vi "SP Format Error Messages.vi"(8 "error in (no error)":errorcluster) -> (0 "error out":errorcluster)   [LabVIEW 2011]
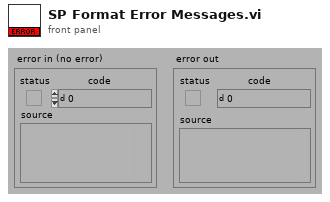
[diagram p1: front panel]
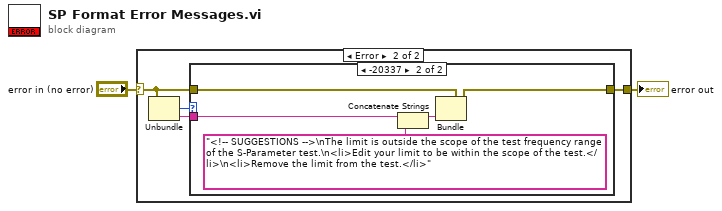
[diagram p0: block diagram]
diagram:
  n1 = case shown="Error" "error in (no error)" {
    selector: "error in (no error)" -> [w3 w5]
    tunnel: [w3 w4] -> w1
    frame No Error {
    }
    frame Error {
      n2 = Unbundle(w5) -> ("code"=w7:i32, "source"=w6:string)  [unwired: 1 out]
      n3 = case shown="-20337" w7 {
        tunnel: w6 -> [_ w13]
        tunnel: w5 -> [w8 w11]
        tunnel: [w8 w9] -> w4
        frame Default {
        }
        frame -20337 {
          n4 = Concatenate Strings(w13, "<!-- SUGGESTIONS -->\nThe limit is outside the scope of the test frequency range of the S-Parameter test.\n<li>Edit your limit to be within the scope of the test.</li>\n<li>Remove the limit from the test.</li>" ("string")) -> (w10:string)
          n5 = Bundle(cluster=w11, "source"=w10) -> (w9:errorcluster)  [unwired: 2 out]
        }
      }
    }
  }
  "error out" <- w1
